vi "quantity.vi"() -> ()   [LabVIEW 2013]
panel:
  in  "set all unc to value of first":bool
  out "Waveform Graph":dbl[](graph)
  in  "Array 3":dbl[](array[numeric])
  in  "Numeric 2":dbl
  in  "Numeric":dbl
  in  "Array":dbl[](array[numeric])
  # "GENERATE"
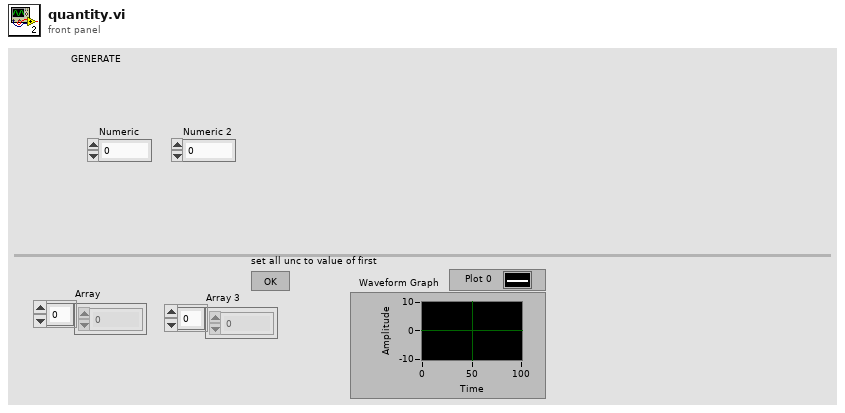
[diagram p1: front panel]
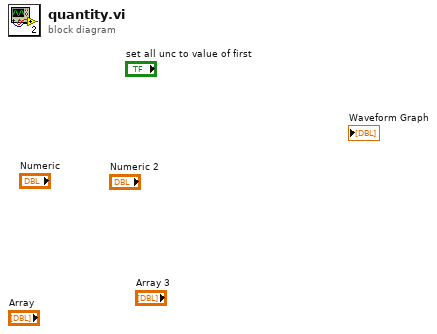
[diagram p0: block diagram]
diagram:
